vi "rename_document.vi"(0 "Device In":T1, 5 "New Name":string, 11 "error in":errorcluster) -> (4 "Device Out":T1, 6 "Comm":T2, 15 "error out":errorcluster)   [LabVIEW 2019]
uses:
  <userlib>/IoT Devices/_subVIs/HTTPComm.ctl
  _SubVI/Cluster.ctl
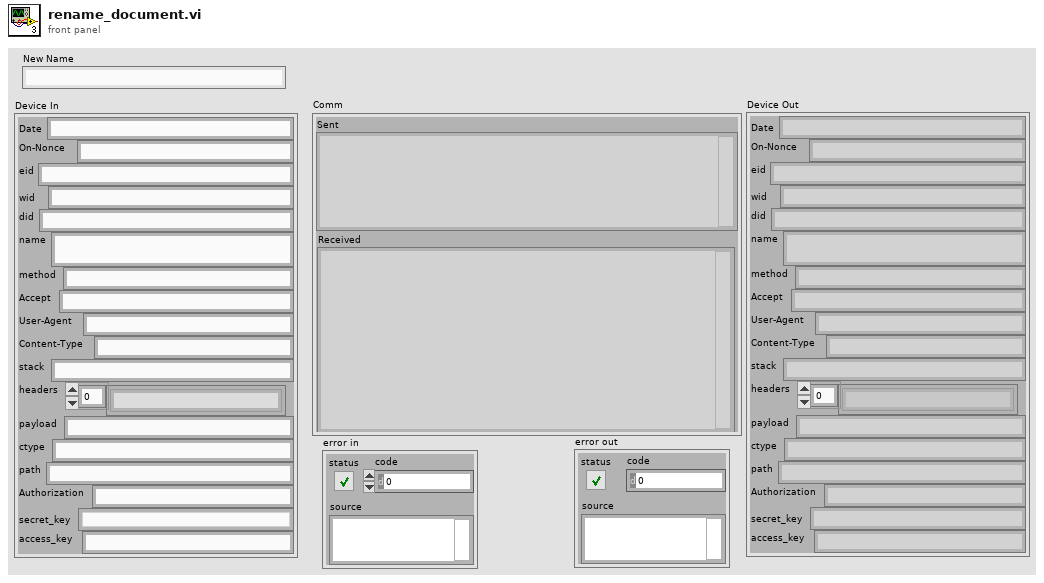
[diagram p1: front panel]
types:
  T1 = typedef "Cluster.ctl" = cluster{"Date":string, "On-Nonce":string, "eid":string, "wid":string, "did":string, "name":string, "method":string, "Accept":string, "User-Agent":string, "Content-Type":string, "stack":string, "headers":string[], "payload":string, "ctype":string, "path":string, "Authorization":string, "secret_key":string, "access_key":string}
  T2 = typedef "HTTPComm.ctl" = cluster{"url":string, "sent headers":string, "sent body":string, "headers":string, "body":string, "Sent":string, "Received":string}
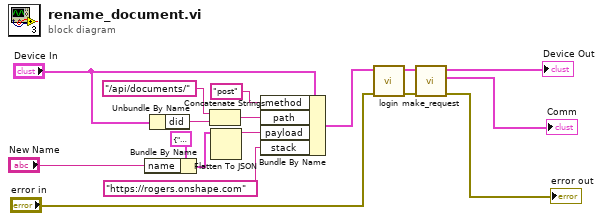
[diagram p0: block diagram]
diagram:
  n1 = Bundle By Name(cluster=cluster{"name":string} {"name"="milan"}, "name"="New Name") -> (w15:cluster{"name":string})
  n2 = Unbundle By Name("Device In") -> ("did"=w4:string)
  n3 = Concatenate Strings("/api/documents/" ("payload"), w4) -> (w12:string)
  n4 = Flatten To JSON(anything=w15) -> (JSON string=w11:string)  [unwired: 2 in, 1 out]
  n5 = Bundle By Name(cluster="Device In", "method"="post" ("Method"), "path"=w12, "payload"=w11, "stack"="https://rogers.onshape.com" ("stacks")) -> (w2:T1)
  n6 = call "login.vi"("error in"="error in", "Device In"=w2) -> ("error out"=w7:errorcluster, "Device Out"=w8:T1)  [unwired: 8 in]
  n7 = call "make_request.vi"("Error in"=w7, "Device In"=w8) -> ("error out"=→"error out":errorcluster, "Comm"=→"Comm":T2, "Device Out"=→"Device Out":T1)  [unwired: 7 in]
